vi "ActionVIOnCompile.vi"(8 "error in (no error)":errorcluster, 11 "Device Item Ref in":T1 format="%.0x") -> (0 "error out":errorcluster)   [LabVIEW 2015, in "Inline Async Example System Explorer.lvlib"]
uses:
  Inline Async Example System Explorer.lvlib
  <vilib>/NI Veristand/Custom Device API/Custom Device Item Ref.ctl
  <vilib>/NI Veristand/Custom Device Tools/Custom Device Utility Library/NI VeriStand - Search for Item by Name.vi
  <vilib>/NI Veristand/Custom Device API/Set Item Property (Variant).vi
  <vilib>/NI Veristand/Custom Device Tools/Custom Device Utility Library/Custom Device Utility Library.lvlib
  <vilib>/NI Veristand/Custom Device API/Custom Device API.lvlib
  Inline Async APIs/Data Access System Explorer/Data Access System Explorer.lvlib
panel:
  in  "Boolean":bool
  out "error out 3":errorcluster
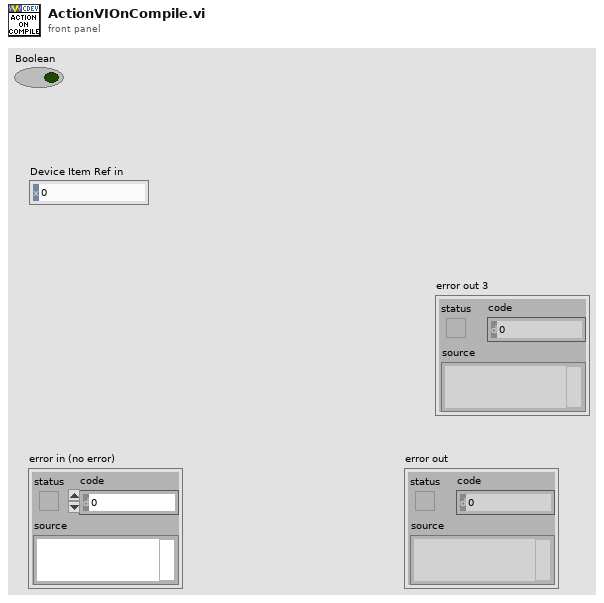
[diagram p1: front panel]
types:
  T1 = typedef "Custom Device API.lvlib/Custom Device Item Ref.ctl" = u64
  T2 = enum16{"Output/Write", "Input/Read", "Input/ReadWrite"}
  T3 = cluster{"Name":string, "Type":enum16{"Output/Write", "Input/Read", "Input/ReadWrite"}, "VS Refs":T1[]}
  T4 = typedef "Custom Device API.lvlib/Custom Device Item Info.ctl" = cluster{"Name":string, "Is Channel":bool, "GUID":string, "Is Waveform":bool}
  T5 = cluster{"Name":string, "Type":enum16{"Output/Write", "Input/Read", "Input/ReadWrite"}, "VS Refs":T1[]}[]
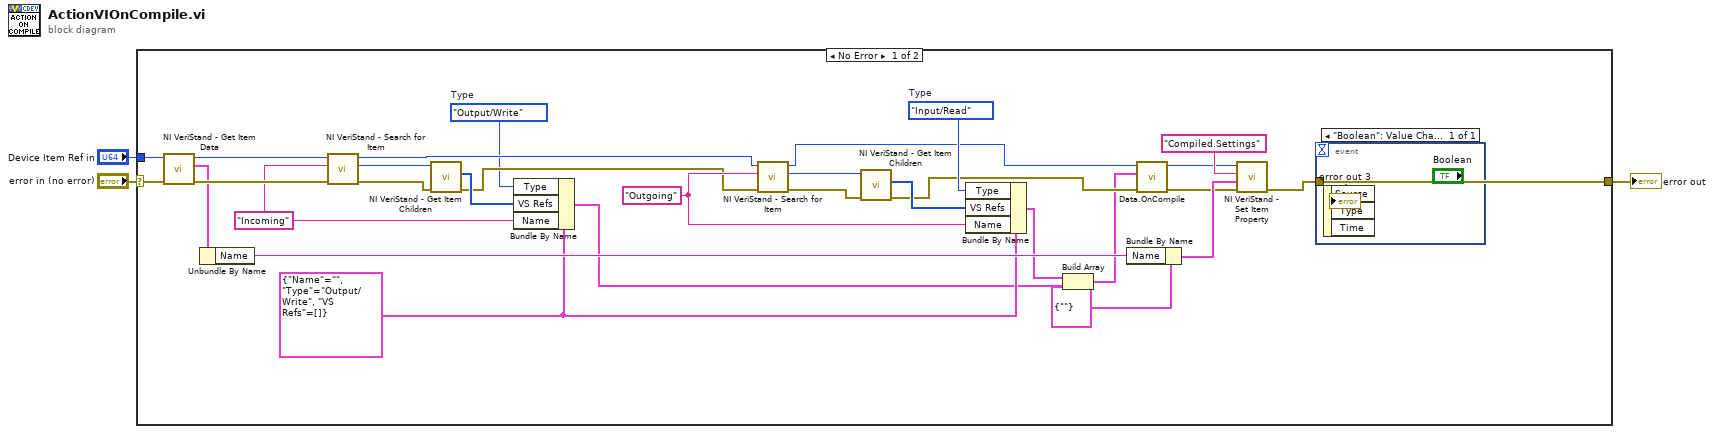
[diagram p0: block diagram]
diagram:
  n1 = case shown="No Error" "error in (no error)" {
    selector: "error in (no error)" -> [w25 w35]
    tunnel: [w26 w35] -> w2
    tunnel: "Device Item Ref in" -> [w24 _]
    frame No Error {
      w10 = T2."Input/Read"  # Type
      w11 = T2."Output/Write"  # Type
      w16 = T3 {"Name"="", "Type"=enum."Output/Write", "VS Refs"=[]} ("Group")
      w17 = "Outgoing" ("Item Name")
      w19 = "Incoming" ("Item Name")
      n2 = call <vilib>:"NI VeriStand - Get Item Data.vi"("error in (no error)"=w25, "Item Ref in"=w24) -> ("error out"=w22:errorcluster, "Item Info"=w21:T4, "Item Ref out"=w23:T1)  [unwired: 6 in, 1 out]
      n3 = Unbundle By Name(w21) -> ("Name"=w20:string)
      n4 = call-poly <vilib>:"NI VeriStand - Search for Item.vi"("error in"=w22, "Item Name"=w19, "Section Ref in"=w23) -> ("error out"=w33:errorcluster, "Item Ref"=w32:T1, "Section Ref out"=w12:T1)  [unwired: 5 in, 1 out]
      n5 = call <vilib>:"NI VeriStand - Get Item Children.vi"("error in (no error)"=w33, "Item Ref in"=w32) -> ("error out"=w13:errorcluster, "Child Refs"=w18:T1[])  [unwired: 6 in, 2 out]
      n6 = Bundle By Name(cluster=w16, "Type"=w11, "VS Refs"=w18, "Name"=w19) -> (w15:T3)
      n7 = call-poly <vilib>:"NI VeriStand - Search for Item.vi"("error in"=w13, "Item Name"=w17, "Section Ref in"=w12) -> ("error out"=w30:errorcluster, "Item Ref"=w31:T1, "Section Ref out"=w6:T1)  [unwired: 5 in, 1 out]
      n8 = call <vilib>:"NI VeriStand - Get Item Children.vi"("error in (no error)"=w30, "Item Ref in"=w31) -> ("error out"=w8:errorcluster, "Child Refs"=w9:T1[])  [unwired: 6 in, 2 out]
      n9 = Bundle By Name(cluster=w16, "Type"=w10, "VS Refs"=w9, "Name"=w17) -> (w14:T3)
      n10 = Build Array(w14, w15) -> (w4:T5)
      n11 = Bundle By Name(cluster=cluster{"Name":string} {"Name"=""}, "Name"=w20) -> (w27:cluster{"Name":string})
      n12 = call "Data.OnCompile.vi"("error in"=w8, "VS Ref Groups"=w4, "Custom Device Ref"=w6) -> ("error out"=w7:errorcluster, "Custom Device Ref"=w5:T1)  [unwired: 7 in]
      n13 = call-poly <vilib>:"NI VeriStand - Set Item Property.vi"("error in (no error)"=w7, "Value"=w27, "Property Name"="Compiled.Settings", "Item Ref in"=w5) -> ("error out"=w26:errorcluster)  [unwired: 5 in, 2 out]
      n14 = event shown="[0] \"Boolean\": Value Change" {
        selector: _ -> [_]
        dyn-events: _ -> [_]
        timeout: _ -> [_]
        tunnel: w26 -> [w34]
        event "Boolean": Value Change {
          n15 = event-data() -> ()  [unwired: 1 in, 3 out]
          "error out 3" <- w34
        }
      }
    }
    frame Error {
    }
  }
  "error out" <- w2
